vi "dispense test.vi"() -> ()   [LabVIEW 2020]
uses:
  Controller/Dispenser/Dispenser.lvclass
  Controller/Controller.lvclass
panel:
  in  "pressure":dbl
  in  "on/off":bool
  in  "stop":bool
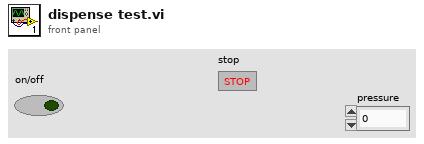
[diagram p1: front panel]
types:
  T1 = typedef "Controller.lvclass/Controllers.ctl" = cluster{"I-O.lvclass":refnum<class "I-O.lvclass">, "Dispenser.lvclass":refnum<class "Dispenser.lvclass">, "Gantry":refnum<k24>}
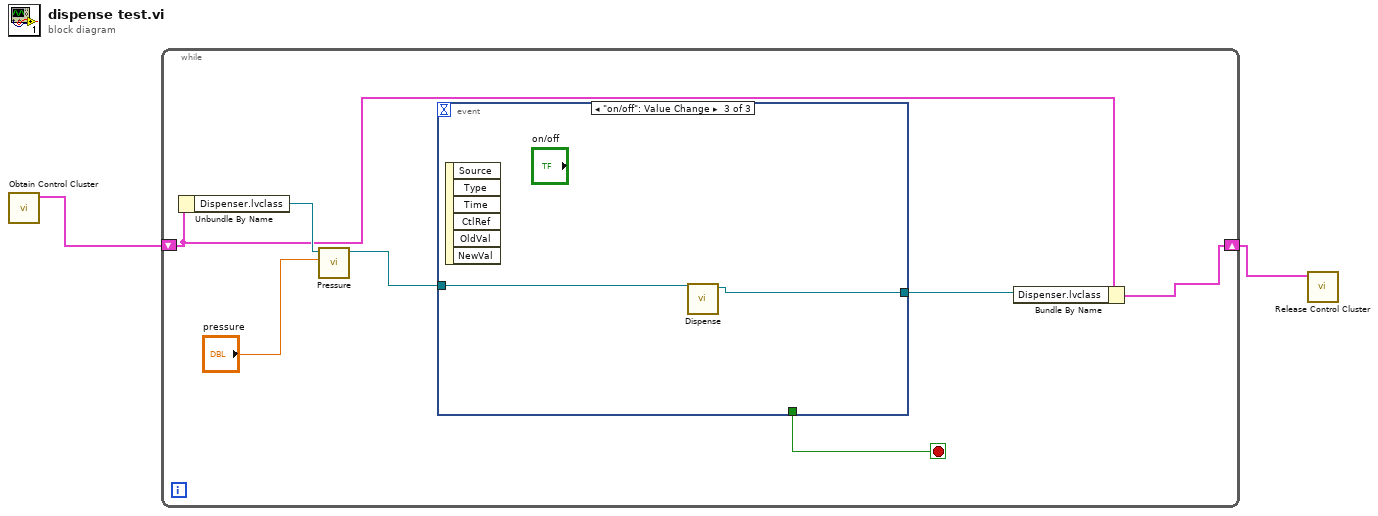
[diagram p0: block diagram]
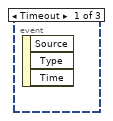
[diagram p2: hidden frame]
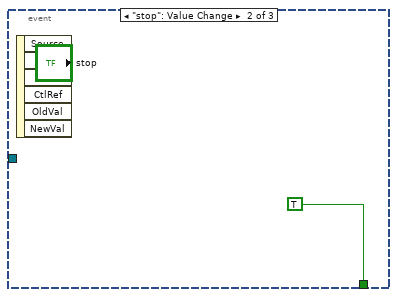
[diagram p3: hidden frame]
diagram:
  n1 = call "Obtain Control Cluster.vi"() -> ("Control Out"=w2:T1)  [unwired: 11 in]
  n2 = while {
    shift-right: [w3] -> w1
    shift-left: w2 -> [w5]
    stop <- w9 stop-if-true
    n3 = Unbundle By Name(w5) -> ("Dispenser.lvclass"=w8:refnum<class "Dispenser.lvclass">)
    n4 = call-dynamic "Pressure.vi"("Pressure"="pressure", "Dispenser in"=w8) -> ("Dispenser out"=w6:refnum<class "Dispenser.lvclass">)  [unwired: 8 in, 1 out]
    n5 = event shown="[2] \"on/off\": Value Change" {
      selector: _ -> [_ _ _]
      dyn-events: _ -> [_ _ _]
      timeout: _ -> [_ _ _]
      tunnel: [_ TRUE _] -> w9
      tunnel: w6 -> [_ _ w12]
      tunnel: [_ _ w11] -> w4
      event Timeout {
        n6 = event-data() -> ()  [unwired: 1 in, 3 out]
      }
      event "stop": Value Change {
        n7 = event-data() -> ()  [unwired: 1 in, 6 out]
      }
      event "on/off": Value Change {
        n8 = event-data() -> ()  [unwired: 1 in, 6 out]
        n9 = call-dynamic "Dispense.vi"("Dispenser in"=w12) -> ("Dispenser out"=w11:refnum<class "Dispenser.lvclass">)  [unwired: 9 in, 1 out]
      }
    }
    n10 = Bundle By Name(cluster=w5, "Dispenser.lvclass"=w4) -> (w3:T1)
  }
  n11 = call "Release Control Cluster.vi"("output cluster"=w1) -> ()  [unwired: 11 in]
